vi "Read ADC.vi"(8 "error in (no error)":errorcluster, 10 "Channel":i32, 11 "UI ACTOR in":refnum<class "UI ACTOR.lvclass">) -> (0 "error out":errorcluster, 3 "UI ACTOR out":refnum<class "UI ACTOR.lvclass">)   [LabVIEW 2020, in "UI ACTOR.lvlib" / "UI ACTOR.lvclass"]
uses:
  UI ACTOR.lvclass
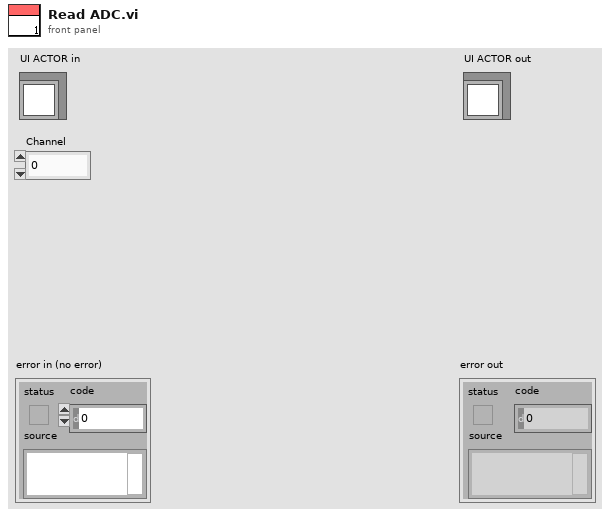
[diagram p1: front panel]
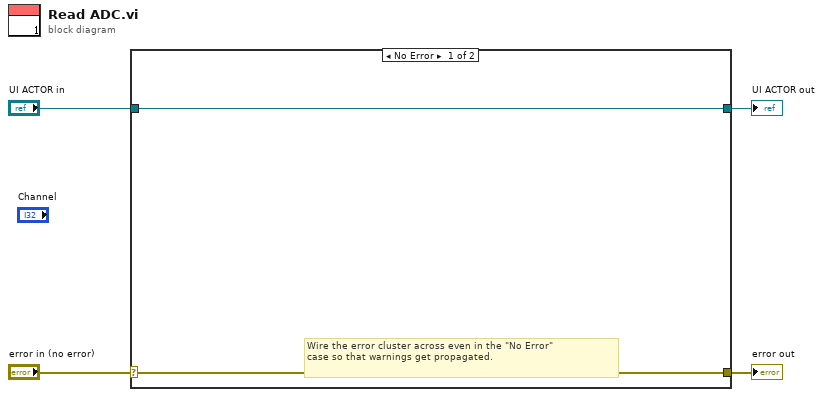
[diagram p0: block diagram]
diagram:
  n1 = case shown="No Error" "error in (no error)" {
    selector: "error in (no error)" -> [w5 w8]
    tunnel: [w5 w8] -> w3
    tunnel: [w6 w7] -> w1
    tunnel: "UI ACTOR in" -> [w6 w7]
    frame No Error {
      # "Wire the error cluster across even in the \"No Error\"\ncase so that warnings get propagated."
    }
    frame Error {
    }
  }
  "error out" <- w3
  "UI ACTOR out" <- w1
